vi "FailureDescription.vi"(8 "error in (no error)":errorcluster, 10 "Actual":variant, 11 "Constraint in":refnum<class "Constraint.lvclass">) -> (0 "error out":errorcluster, 2 "Failure Description":string, 3 "Constraint out":refnum<class "Constraint.lvclass">)   [LabVIEW 2017, in "Transparent Assertions.lvlib" / "Constraints.lvlib" / "Constraint.lvclass"]
doc: "Return the second part of the scentence \"Failed asserting that ...\""
uses:
  Constraint.lvclass
  <vilib>/PNR/JSONtext Object Serialization/Generic Object Serializer/Generic Object Serializer.lvclass
  C:/Program Files/National Instruments/LabVIEW 2017/vi.lib/JDP Science/JSONtext/LVClass Serializer/JSONtext LVClass Serializer.lvclass
  <vilib>/PNR/JSONtext Object Serialization/Generic Object Serializer/Type Name Handling.ctl
  <vilib>/PNR/JSONtext Object Serialization/Generic Object Serializer/Generic Object Serializer.lvclass/Generic Object Serializer.ctl
  b2f06bc6-85a8-4a2f-8cfc-0c2be206f2da.vi
  <vilib>/PNR/JSONtext Object Serialization/Generic Object Serializer/Write Type Name Handling.vi
  <vilib>/JDP Science/JSONtext/Variant to JSON Text.vi
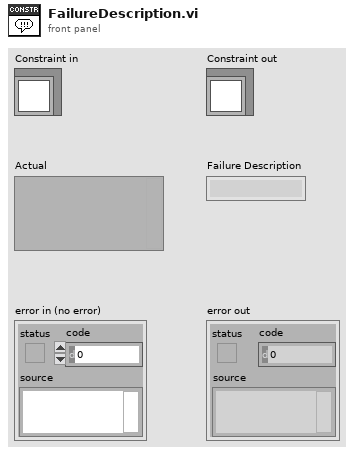
[diagram p1: front panel]
types:
  T1 = typedef "Generic Object Serializer.lvclass/Type Name Handling.ctl" = enum16{"None", "Inline"}
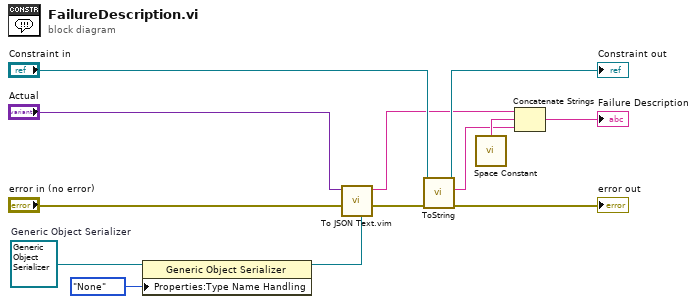
[diagram p0: block diagram]
diagram:
  w2 = refnum<class "Generic Object Serializer.lvclass"> refnum  # Generic Object Serializer
  n1 = property class="Generic Object Serializer"(reference=w2, "Properties:Type Name Handling"=Type_Name_Handling."None" ("Type Name Handling")) -> (reference out=w1:refnum<class "Generic Object Serializer.lvclass">)  [unwired: 1 in, 1 out]
  n2 = call "To JSON Text.vim"("LVClass Serializer"=w1, "error in (no error)"="error in (no error)", "Anything"="Actual") -> ("error out"=w7:errorcluster, "<JSON>"=w5:string)  [unwired: 7 in]
  n3 = call-dynamic "ToString.vi"("error in (no error)"=w7, "Constraint in"="Constraint in") -> ("error out"=→"error out":errorcluster, "String"=w4:string, "Constraint out"=→"Constraint out":refnum<class "Constraint.lvclass">)  [unwired: 7 in]
  n4 = call <vilib>:"Space Constant.vi"() -> ("String"=w6:string)
  n5 = Concatenate Strings(w5, w6, w4) -> (→"Failure Description":string)
